vi "createGoal.vi"(8 "error in (no error)":errorcluster, 9 "Goal.lvclass":refnum<class "Goal.lvclass">, 10 "WhichMonth.lvclass":refnum<class "WhichMonth.lvclass">, 11 "Account History in":refnum<class "Account History.lvclass">) -> (0 "error out":errorcluster, 3 "Account History out":refnum<class "Account History.lvclass">)   [LabVIEW 2018, in "Account History.lvclass"]
uses:
  Account History.lvclass
  WhichMonth/WhichMonth.lvclass
  Goal/Goal.lvclass
  C:/GitRepos/Filthy-Lucre-Budgetizer/source/support/classes/Category/Category.lvclass
  Category/Category.lvclass
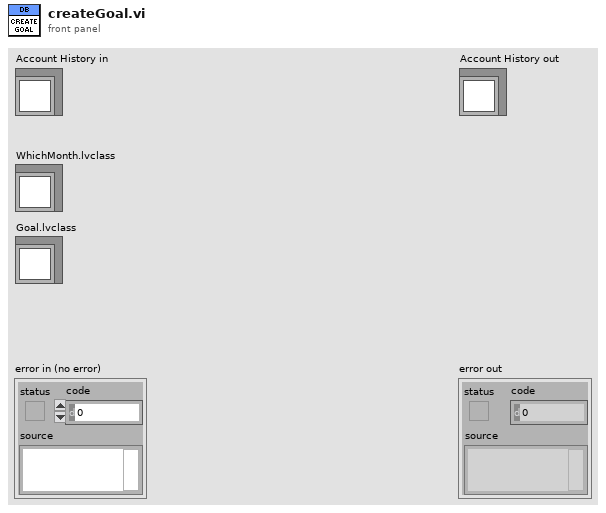
[diagram p1: front panel]
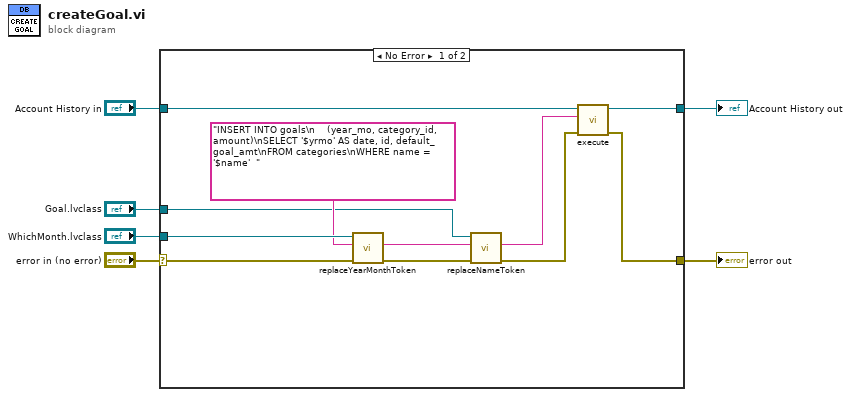
[diagram p0: block diagram]
diagram:
  n1 = case shown="No Error" "error in (no error)" {
    selector: "error in (no error)" -> [w12 w19]
    tunnel: [w15 w19] -> w5
    tunnel: [w16 w18] -> w3
    tunnel: "Account History in" -> [w17 w18]
    tunnel: "WhichMonth.lvclass" -> [w14 _]
    tunnel: "Goal.lvclass" -> [w8 _]
    frame No Error {
      n2 = call "replaceYearMonthToken.vi"("error in (no error)"=w12, "Query In"="INSERT INTO goals\n    (year_mo, category_id, amount)\nSELECT '$yrmo' AS date, id, default_goal_amt\nFROM categories\nWHERE name = '$name'  ", "WhichMonth in"=w14) -> ("error out"=w7:errorcluster, "Query Out"=w9:string)  [unwired: 6 in, 1 out]
      n3 = call "replaceNameToken.vi"("error in (no error)"=w7, "Query In"=w9, "Category in"=w8) -> ("error out"=w11:errorcluster, "Query Out"=w10:string)  [unwired: 6 in, 1 out]
      n4 = call "execute.vi"("error in (no error)"=w11, "SQL query"=w10, "Database in"=w17) -> ("error out"=w15:errorcluster, "Database out"=w16:refnum<class "Account History.lvclass">)  [unwired: 7 in]
    }
    frame Error {
    }
  }
  "error out" <- w5
  "Account History out" <- w3
